vi "gyro launch app V1.vi"() -> ()   [LabVIEW 2020]
uses:
  <vilib>/event_ctls.llb/eventvkey.ctl
  server talk-to-back pair.ctl
  server talkback message type.ctl
  server talkto message type.ctl
  agregator -- action.ctl
  interpolation state - real.ctl
  pll internal user event action.ctl
  launch items list.ctl
  que event bag action.ctl
  cursor action.ctl
  linear interpolation - real.vi
panel:
  in  "Main":enum32{"all", "other"}(tab)
  in  "pll monitor":bool
  in  "sweeper engine":bool=TRUE
  in  "fitter":bool
  in  "source":bool
  in  "exit!":bool=TRUE
  in  "pll engine":bool
  in  "sweeper monitor":bool=TRUE
  out "VKey":T1=enum."Cmd"
  out "Char":i16
  out "Stoped?":bool=TRUE
  out "talking pair array":T2[](array[typedef])
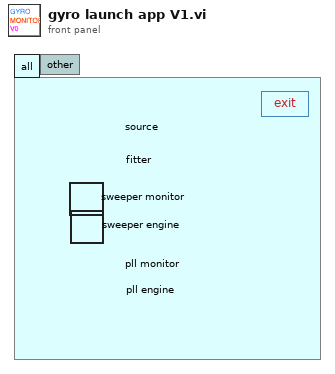
[diagram p1: front panel]
types:
  T1 = typedef "eventvkey.ctl" = enum16{"ASCII", "Enter", "Return", "Shift", "Ctrl", "Alt", "Cmd", "Opt", "Caps", "NumLock", "Clear", "Break", "Up", "Down", "Left", "Right", "Insert", "Delete", "Home", "End", "PageUp", "PageDown", "Escape", "Help", "Pause", "ScrollLock", "F1", "F2", "F3", "F4", "F5", "F6", "F7", "F8", "F9", "F10", "F11", "F12", "F13", "F14", "F15", "F16", "F17", "F18", "F19", "F20", "F21", "F22", "F23", "F24", "Play", "VolumeUp", "VolumeDown", "Mute", "Two Byte Char"}
  T2 = typedef "server talk-to-back pair.ctl" = cluster{"talkback event":refnum<user-event>, "talkto event":refnum<user-event>}
  T3 = typedef "launch items list.ctl" = enum16{"void", "source", "pll engine", "pll monitor", "sweeper engine", "sweeper monitor", "fitter"}
  T4 = typedef "que event bag action.ctl" = enum16{"check", "add", "init"}
  T5 = typedef "server talkback message type.ctl" = cluster{"message":enum16{"new", "void"}}
  T6 = typedef "server talkto message type.ctl" = cluster{"message":enum16{"stop", "start", "update pars", "update request", "new", "launch", "exit", "get", "reset", "pause", "unpause"}}
  T7 = typedef "pll internal user event action.ctl" = enum16{"gear pll engine", "start pll async", "stop pll async", "toggle pll async", "gear sweeper", "start sweeper", "stop sweeper", "toggle sweeper", "accept frequency", "reset lorentzian", "accept lorentzian", "update cursors", "pause pll", "unpause pll", "void", "exit", "gear sweeper monitor", "gear sweeper engine", "gear fitter", "gear sourcer", "gear pll monitor"}
  T8 = typedef "interpolation state - real.ctl" = cluster{"requested size":i32, "Array":dbl[], "actual number of elements":i32}
  T9 = typedef "agregator -- action.ctl" = enum16{"append", "interpolate", "empty!", "force", "init", "scale", "read last"}
  T10 = enum32{"Invalid", "Standard", "Closed", "Hidden", "Minimized", "Maximized"}
  T11 = typedef "cursor action.ctl" = enum16{"range", "read", "write", "check", "zoom out", "smart zoom out", "zoom to aspect ratio 1", "zoom to win", "zoom out 20%", "zoom in 20%", "-empty", "smart zoom out&aspect", "move range left 20%", "move range right 20%", "move range up 20%", "move range down 20%", "zoom to X win", "zoom to Y win", "zoom out X", "zoom out Y", "zoom in X", "zoom in Y", "check plot scale"}
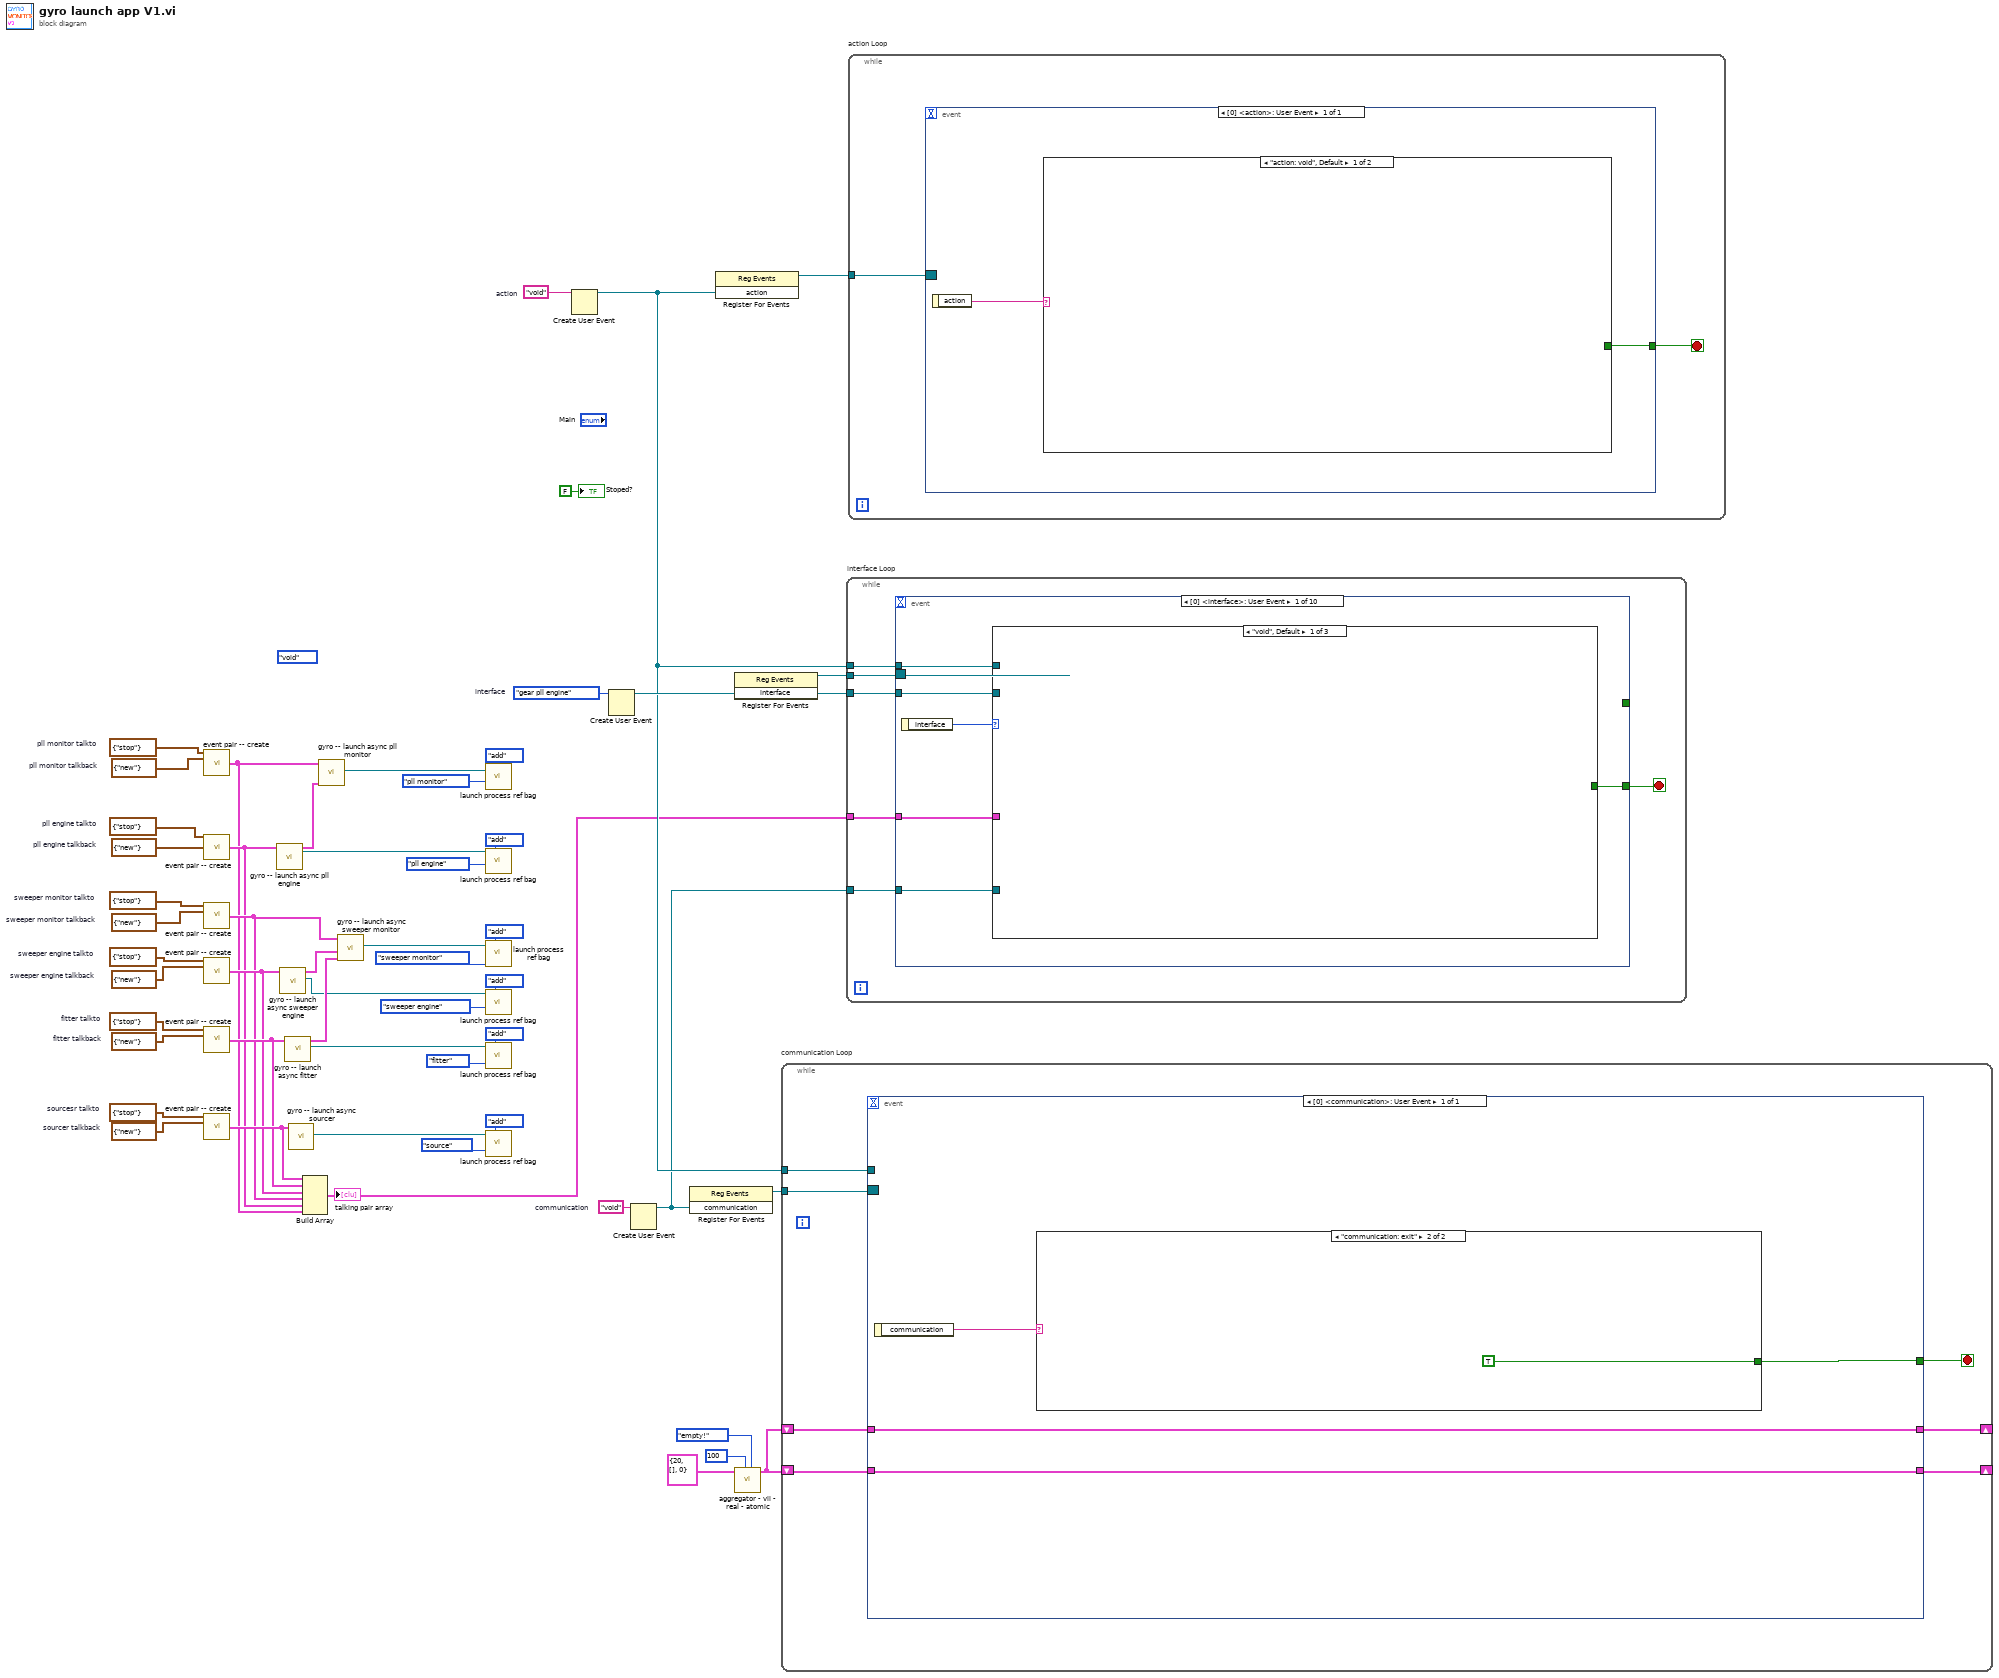
[diagram p0: block diagram]
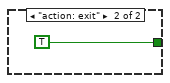
[diagram p2: hidden frame]
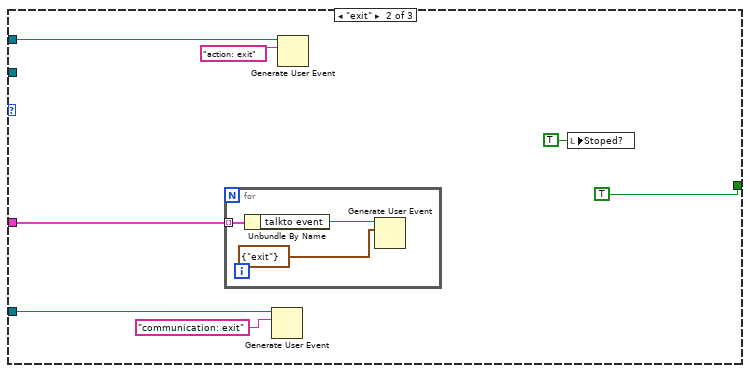
[diagram p4: hidden frame]
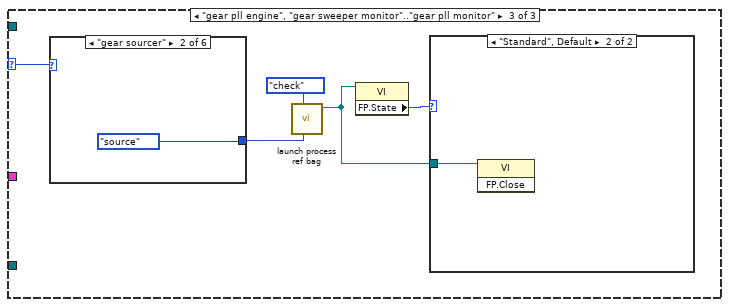
[diagram p5: hidden frame]
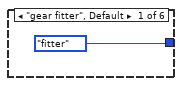
[diagram p6: hidden frame]
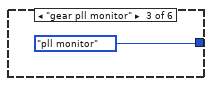
[diagram p7: hidden frame]
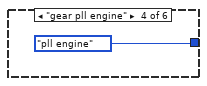
[diagram p8: hidden frame]
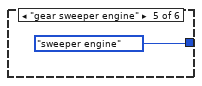
[diagram p9: hidden frame]
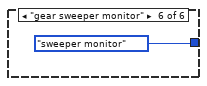
[diagram p10: hidden frame]
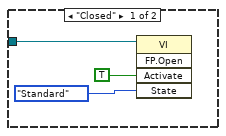
[diagram p11: hidden frame]
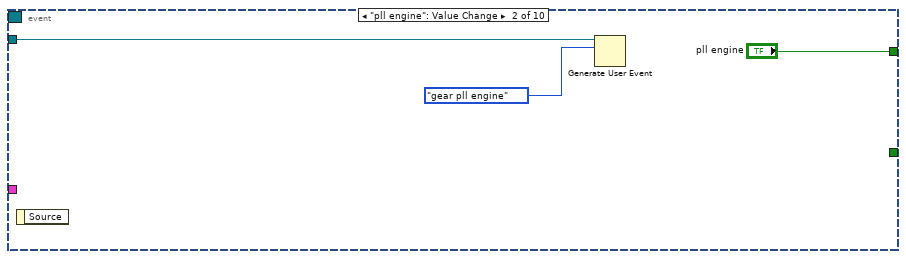
[diagram p12: hidden frame]
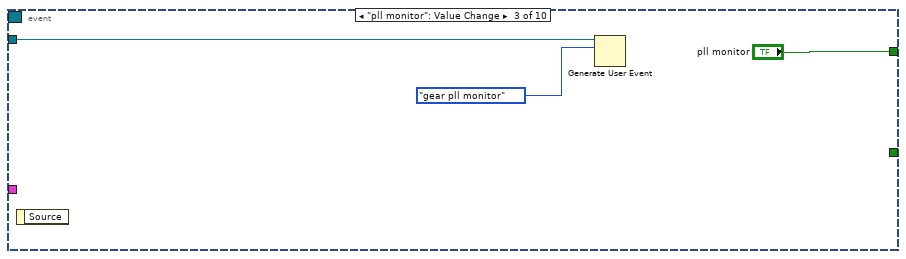
[diagram p13: hidden frame]
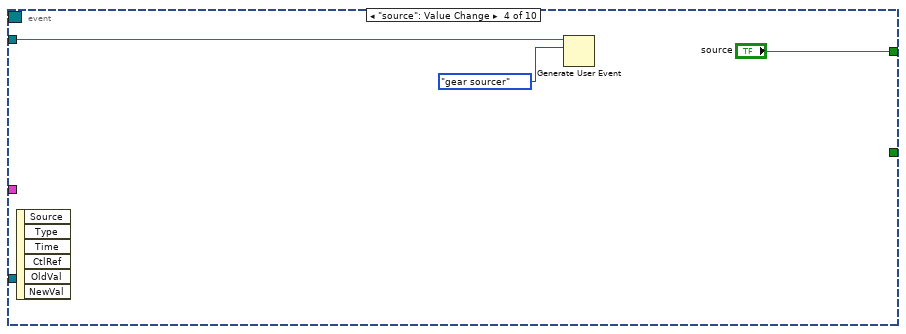
[diagram p14: hidden frame]
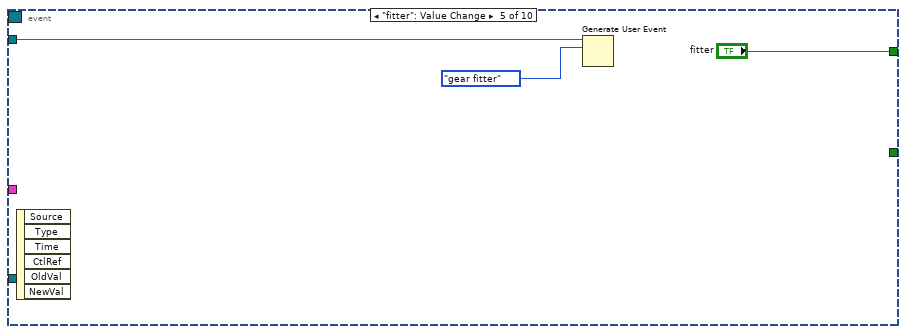
[diagram p15: hidden frame]
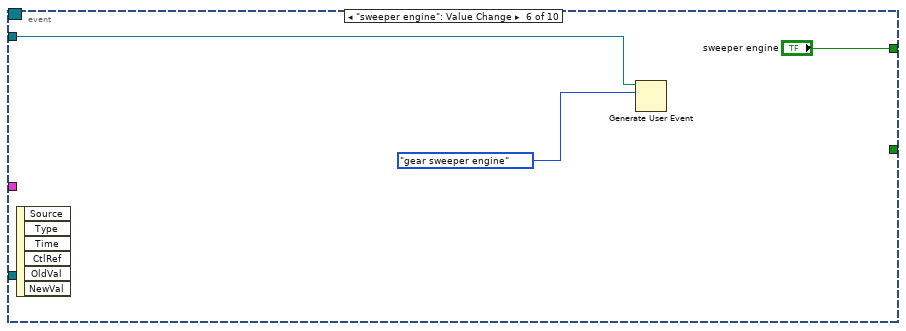
[diagram p16: hidden frame]
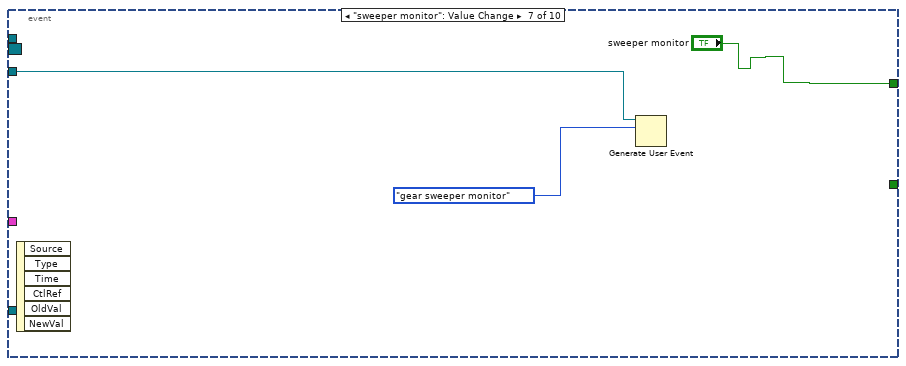
[diagram p17: hidden frame]
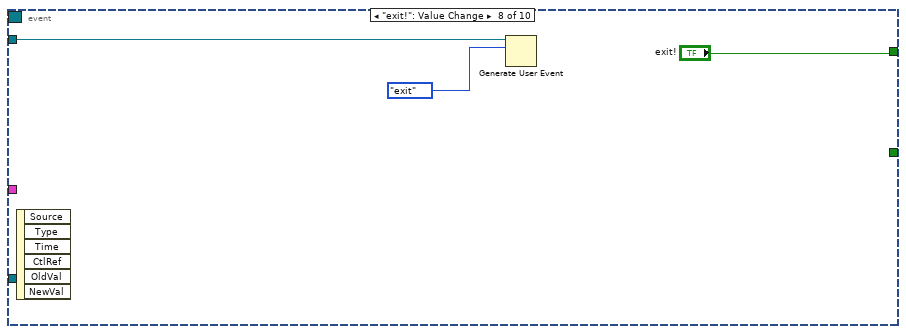
[diagram p18: hidden frame]
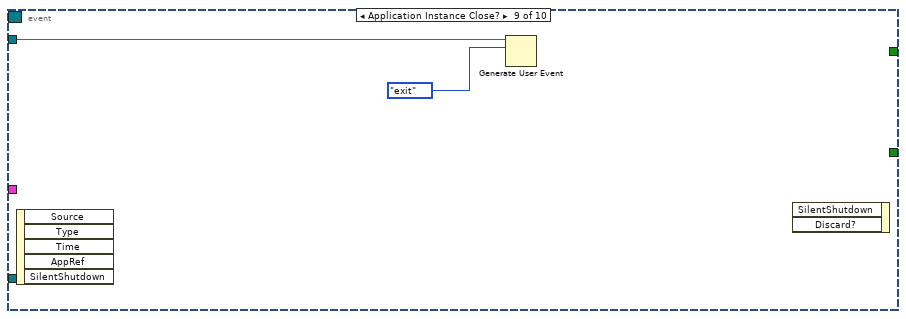
[diagram p19: hidden frame]
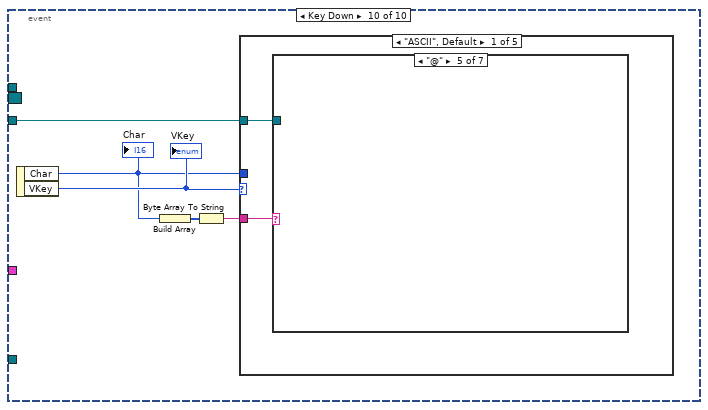
[diagram p20: hidden frame]
diagram:
  (unwired) launch_items_list."void" ("launch items")
  w37 = T5 {"message"=enum."new"}  # pll monitor talkback
  w38 = T6 {"message"=enum."stop"}  # pll monitor talkto
  w41 = "void"  # communication
  w44 = "void"  # action
  w26 = T5 {"message"=enum."new"}  # sourcer talkback
  w27 = T6 {"message"=enum."stop"}  # sourcesr talkto
  w35 = T5 {"message"=enum."new"}  # pll engine talkback
  w36 = T6 {"message"=enum."stop"}  # pll engine talkto
  w33 = T5 {"message"=enum."new"}  # sweeper monitor talkback
  w34 = T6 {"message"=enum."stop"}  # sweeper monitor talkto
  w31 = T5 {"message"=enum."new"}  # sweeper engine talkback
  w32 = T6 {"message"=enum."stop"}  # sweeper engine talkto
  w29 = T5 {"message"=enum."new"}  # fitter talkback
  w30 = T6 {"message"=enum."stop"}  # fitter talkto
  w48 = pll_internal_user_event_action."gear pll engine"  # interface
  n1 = call "event pair -- create.vi"("talkto"=w38, "talkback"=w37) -> ("even pair out"=w19:T2)  [unwired: 11 in, 2 out]
  n2 = call "event pair -- create.vi"("talkto"=w36, "talkback"=w35) -> ("even pair out"=w21:T2)  [unwired: 11 in, 2 out]
  n3 = call "event pair -- create.vi"("talkto"=w34, "talkback"=w33) -> ("even pair out"=w22:T2)  [unwired: 11 in, 2 out]
  n4 = call "event pair -- create.vi"("talkto"=w32, "talkback"=w31) -> ("even pair out"=w23:T2)  [unwired: 11 in, 2 out]
  n5 = call "event pair -- create.vi"("talkto"=w30, "talkback"=w29) -> ("even pair out"=w24:T2)  [unwired: 11 in, 2 out]
  n6 = call "event pair -- create.vi"("talkto"=w27, "talkback"=w26) -> ("even pair out"=w25:T2)  [unwired: 11 in, 2 out]
  n7 = call "gyro -- launch async pll engine.vi"("pll event pair IN"=w21) -> ("reference out"=w13:refnum<vi>, "pll event pair OUT"=w39:T2)  [unwired: 9 in]
  n8 = call "gyro -- launch async sweeper engine.vi"("sweeper event pair"=w23) -> ("reference out"=w7:refnum<vi>, "sweeper event pair OUT"=w47:T2)  [unwired: 9 in]
  n9 = call "gyro -- launch async fitter.vi"("fitter pair"=w24) -> ("reference out"=w4:refnum<vi>, "fitter pair OUT"=w28:T2)  [unwired: 9 in]
  n10 = call "gyro -- launch async sourcer.vi"("sourcer pair"=w25) -> ("reference out"=w1:refnum<vi>)  [unwired: 9 in, 1 out]
  n11 = Build Array(w25, w24, w23, w22, w21, w19) -> (w20:T2[])
  "talking pair array" <- w20
  n12 = call "gyro -- launch async pll monitor.vi"("pll engine pair IN"=w39, "pll monitor event pair IN"=w19) -> ("reference out"=w16:refnum<vi>)  [unwired: 8 in, 1 out]
  n13 = call "gyro -- launch async sweeper monitor.vi"("fitter event pair"=w28, "async sweeper engine event pair"=w47, "sweeper monitor event pair"=w22) -> ("reference out"=w10:refnum<vi>)  [unwired: 8 in]
  n14 = call "launch process ref bag.vi"("launch items"=launch_items_list."pll monitor", "bag action"=que_event_bag_action."add", "process ref IN"=w16) -> ()  [unwired: 8 in, 1 out]
  n15 = call "launch process ref bag.vi"("launch items"=launch_items_list."pll engine", "bag action"=que_event_bag_action."add", "process ref IN"=w13) -> ()  [unwired: 8 in, 1 out]
  n16 = call "launch process ref bag.vi"("launch items"=launch_items_list."sweeper monitor", "bag action"=que_event_bag_action."add", "process ref IN"=w10) -> ()  [unwired: 8 in, 1 out]
  n17 = call "launch process ref bag.vi"("launch items"=launch_items_list."sweeper engine", "bag action"=que_event_bag_action."add", "process ref IN"=w7) -> ()  [unwired: 8 in, 1 out]
  n18 = call "launch process ref bag.vi"("launch items"=launch_items_list."fitter", "bag action"=que_event_bag_action."add", "process ref IN"=w4) -> ()  [unwired: 8 in, 1 out]
  n19 = call "launch process ref bag.vi"("launch items"=launch_items_list."source", "bag action"=que_event_bag_action."add", "process ref IN"=w1) -> ()  [unwired: 8 in, 1 out]
  n20 = Create User Event(user event datatype=w44) -> (user event=w42:refnum<user-event>)  [unwired: 1 in, 1 out]
  n21 = Create User Event(user event datatype=w48) -> (user event=w46:refnum<user-event>)  [unwired: 1 in, 1 out]
  n22 = Create User Event(user event datatype=w41) -> (user event=w40:refnum<user-event>)  [unwired: 1 in, 1 out]
  n23 = register-events(w40) -> (reference out=w49:refnum<event-registration>)  [unwired: 2 in, 1 out]
  n24 = register-events(w42) -> (reference out=w43:refnum<event-registration>)  [unwired: 2 in, 1 out]
  n25 = register-events(w46) -> (reference out=w54:refnum<event-registration>)  [unwired: 2 in, 1 out]
  n26 = call "aggregator - vii - real - atomic.vi"("aggregator action"=agregator_--_action."empty!", "requested size"=100, "state IN"=T8 {"requested size"=20, "Array"=[], "actual number of elements"=0}) -> ("state OUT"=w50:T8)  [unwired: 5 in, 3 out]
  n27 = while "communication Loop" {
    shift-right: [w58] -> _
    shift-left: w50 -> [w61]
    shift-right: [w59] -> _
    shift-left: w50 -> [w60]
    tunnel: w49 -> [w57]
    tunnel: w42 -> [w56]
    stop <- w55 stop-if-true
    n28 = event shown="[0] <communication>: User Event" {
      selector: w57 -> [_]
      dyn-events: _ -> [_]
      timeout: _ -> [_]
      tunnel: w61 -> [w63]
      tunnel: w60 -> [w62]
      tunnel: [w62] -> w59
      tunnel: [w63] -> w58
      tunnel: w56 -> [_]
      tunnel: [w64] -> w55
      event User Event {
        n29 = event-data() -> ("communication"=w65:string)  [unwired: 1 in]
        n30 = case shown="\"communication: exit\"" w65 {
          tunnel: [_ TRUE] -> w64
          frame "void", Default {
          }
          frame "communication: exit" {
          }
        }
      }
    }
  }
  n31 = while "interface Loop" {
    tunnel: w54 -> [w72]
    tunnel: w46 -> [w71]
    tunnel: w42 -> [w69]
    tunnel: w40 -> [w68]
    tunnel: w20 -> [w67]
    stop <- w70 stop-if-true
    n32 = event shown="[0] <interface>: User Event" {
      selector: w72 -> [_ _ _ _ _ _ _ _ _ _]
      dyn-events: _ -> [_ _ _ _ _ _ _ _ _ _]
      timeout: _ -> [_ _ _ _ _ _ _ _ _ _]
      tunnel: [_ "pll engine" "pll monitor" "source" "fitter" "sweeper engine" "sweeper monitor" "exit!" _ _] -> _
      tunnel: w71 -> [w77 w106 w109 w112 w115 w118 w121 w123 w126 w127]
      tunnel: [w76 _ _ _ _ _ _ _ _ _] -> w70
      tunnel: w69 -> [w75 _ _ _ _ _ _ _ _ _]
      tunnel: w68 -> [w74 _ _ _ _ _ _ _ _ _]
      tunnel: w67 -> [w73 _ _ _ _ _ _ _ _ _]
      event User Event {
        n33 = event-data() -> ("interface"=w78:T7)  [unwired: 1 in]
        n34 = case shown="\"void\", Default" w78 {
          selector: w78 -> [_ _ w90]
          tunnel: w77 -> [_ _ _]
          tunnel: [_ TRUE _] -> w76
          tunnel: w75 -> [_ w83 _]
          tunnel: w74 -> [_ w80 _]
          tunnel: w73 -> [_ w79 _]
          frame "void", Default {
          }
          frame "exit" {
            n35 = for {
              tunnel: w79 -> [w87] mode=indexing
              n36 = Unbundle By Name(w87) -> ("talkto event"=w86:refnum<user-event>)
              n37 = Generate User Event(user event=w86, event data cluster=T6 {"message"=enum."exit"} ("event data")) -> ()  [unwired: 2 in, 2 out]
            }
            n38 = Generate User Event(user event=w80, event data cluster="communication: exit" ("event data")) -> ()  [unwired: 2 in, 2 out]
            n39 = Generate User Event(user event=w83, event data cluster="action: exit" ("event data")) -> ()  [unwired: 2 in, 2 out]
            n40 = local write "Stoped?"(TRUE ("Stoped?")) -> ()
          }
          frame "gear pll engine", "gear sweeper monitor".."gear pll monitor" {
            n41 = case shown="\"gear sourcer\"" w90 {
              tunnel: [launch_items_list."fitter" ("launch items") launch_items_list."source" ("launch items") launch_items_list."pll monitor" ("launch items") launch_items_list."pll engine" ("launch items") launch_items_list."sweeper engine" ("launch items") launch_items_list."sweeper monitor" ("launch items")] -> w89
              frame "gear fitter", Default {
              }
              frame "gear sourcer" {
              }
              frame "gear pll monitor" {
              }
              frame "gear pll engine" {
              }
              frame "gear sweeper engine" {
              }
              frame "gear sweeper monitor" {
              }
            }
            n42 = call "launch process ref bag.vi"("launch items"=w89, "bag action"=que_event_bag_action."check") -> ("process ref OUT"=w91:refnum<vi>)  [unwired: 9 in]
            n43 = property class="VI"(reference=w91) -> ("FP.State"=w93:T10)  [unwired: 1 in, 2 out]
            n44 = case shown="\"Standard\", Default" w93 {
              tunnel: w91 -> [w102 w103]
              frame "Closed" {
                n45 = invoke class="VI" method="FP.Open"(reference=w102, "Activate"=TRUE ("Activate?"), "State"=T10."Standard" ("Front Panel Window:State")) -> ()  [unwired: 2 in, 5 out]
              }
              frame "Standard", Default {
                n46 = invoke class="VI" method="FP.Close"(reference=w103) -> ()  [unwired: 2 in, 3 out]
              }
            }
          }
        }
      }
      event "pll engine": Value Change {
        n47 = event-data() -> ()  [unwired: 1 in, 1 out]
        n48 = Generate User Event(user event=w106, event data cluster=pll_internal_user_event_action."gear pll engine" ("event data")) -> ()  [unwired: 2 in, 2 out]
      }
      event "pll monitor": Value Change {
        n49 = event-data() -> ()  [unwired: 1 in, 1 out]
        n50 = Generate User Event(user event=w109, event data cluster=pll_internal_user_event_action."gear pll monitor" ("event data")) -> ()  [unwired: 2 in, 2 out]
      }
      event "source": Value Change {
        n51 = event-data() -> ()  [unwired: 1 in, 6 out]
        n52 = Generate User Event(user event=w112, event data cluster=pll_internal_user_event_action."gear sourcer" ("event data")) -> ()  [unwired: 2 in, 2 out]
      }
      event "fitter": Value Change {
        n53 = event-data() -> ()  [unwired: 1 in, 6 out]
        n54 = Generate User Event(user event=w115, event data cluster=pll_internal_user_event_action."gear fitter" ("event data")) -> ()  [unwired: 2 in, 2 out]
      }
      event "sweeper engine": Value Change {
        n55 = event-data() -> ()  [unwired: 1 in, 6 out]
        n56 = Generate User Event(user event=w118, event data cluster=pll_internal_user_event_action."gear sweeper engine" ("event data")) -> ()  [unwired: 2 in, 2 out]
      }
      event "sweeper monitor": Value Change {
        n57 = event-data() -> ()  [unwired: 1 in, 6 out]
        n58 = Generate User Event(user event=w121, event data cluster=pll_internal_user_event_action."gear sweeper monitor" ("event data")) -> ()  [unwired: 2 in, 2 out]
      }
      event "exit!": Value Change {
        n59 = event-data() -> ()  [unwired: 1 in, 6 out]
        n60 = Generate User Event(user event=w123, event data cluster=pll_internal_user_event_action."exit" ("event data")) -> ()  [unwired: 2 in, 2 out]
      }
      event Application Instance Close? {
        n61 = event-data() -> ()  [unwired: 1 in, 5 out]
        n62 = Generate User Event(user event=w126, event data cluster=pll_internal_user_event_action."exit" ("event data")) -> ()  [unwired: 2 in, 2 out]
        n63 = event-data() -> ()  [unwired: 3 in, 1 out]
      }
      event Key Down {
        n64 = event-data() -> ("Char"=w129:i16, "VKey"=w131:T1)  [unwired: 1 in]
        "Char" <- w129
        "VKey" <- w131
        n65 = Build Array(w129) -> (w130:i16[])
        n66 = Byte Array To String(unsigned byte array=w130) -> (string=w128:string)
        n67 = case shown="\"ASCII\", Default" w131 {
          selector: w131 -> [_ _ _ _ w140]
          tunnel: w129 -> [_ _ _ _ _]
          tunnel: w128 -> [w133 _ _ _ _]
          tunnel: w127 -> [w132 _ _ _ _]
          frame "ASCII", Default {
            n68 = case shown="\"@\"" w133 {
              selector: w133 -> [_ w134 _ _ _ _ _]
              tunnel: w132 -> [_ _ _ _ _ _ _]
              frame "0", Default {
              }
              frame "<", ">", "?", "A", "z" {
                n69 = case shown="\"A\"" w134 {
                  tunnel: [cursor_action."zoom out 20%" ("cursor action") cursor_action."zoom in 20%" ("cursor action") cursor_action."smart zoom out&aspect" ("cursor action") cursor_action."smart zoom out" ("cursor action") cursor_action."zoom to aspect ratio 1" ("cursor action")] -> _
                  frame ">" {
                  }
                  frame "<" {
                  }
                  frame "?" {
                  }
                  frame "A" {
                  }
                  frame "z", Default {
                  }
                }
              }
              frame "r" {
              }
              frame "'", ";", "[", "]", "{", "}" {
              }
              frame "@" {
              }
              frame "#" {
              }
              frame "q" {
              }
            }
          }
          frame "Escape" {
          }
          frame "PageUp" {
          }
          frame "PageDown" {
          }
          frame "Up".."Right" {
            n70 = case shown="\"Down\"" w140 {
              tunnel: [cursor_action."move range right 20%" ("cursor action") cursor_action."move range left 20%" ("cursor action") cursor_action."move range up 20%" ("cursor action") cursor_action."move range down 20%" ("cursor action")] -> _
              frame "Right", Default {
              }
              frame "Left" {
              }
              frame "Up" {
              }
              frame "Down" {
              }
            }
          }
        }
      }
    }
  }
  n71 = while "action Loop" {
    tunnel: w43 -> [w146]
    stop <- w145 stop-if-true
    n72 = event shown="[0] <action>: User Event" {
      selector: w146 -> [_]
      dyn-events: _ -> [_]
      timeout: _ -> [_]
      tunnel: [w147] -> w145
      event User Event {
        n73 = event-data() -> ("action"=w148:string)  [unwired: 1 in]
        n74 = case shown="\"action: void\", Default" w148 {
          tunnel: [_ TRUE] -> w147
          frame "action: void", Default {
          }
          frame "action: exit" {
          }
        }
      }
    }
  }
  "Stoped?" <- FALSE ("Stoped?")
